vi "Fluke Calibrator.vi"(8 "error in (no error)":errorcluster, 11 "Fluke Calibrator in":refnum<class "Fluke Calibrator.lvclass">) -> (0 "error out":errorcluster, 3 "Fluke Calibrator out":refnum<class "Fluke Calibrator.lvclass">)   [LabVIEW 2012, in "Fluke Calibrator.lvclass"]
uses:
  Fluke Calibrator.lvclass
  Global/GPIB Numbers.vi
  Utility Classes/Readable/Readable.lvclass
panel:
  out "Status":string
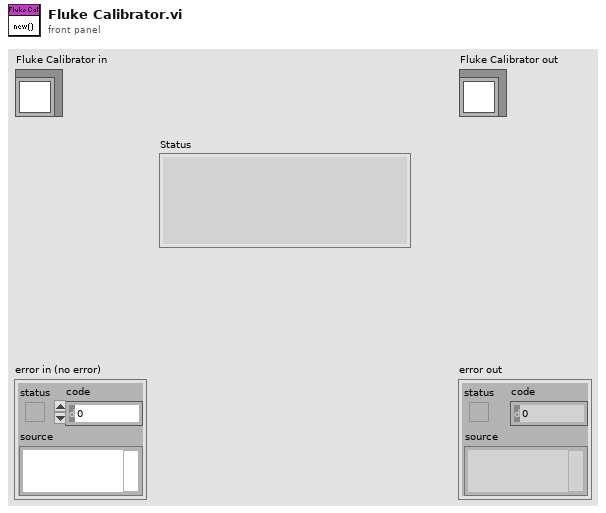
[diagram p1: front panel]
types:
  T1 = typedef "GPIB Type Def.ctl" = cluster{"Name":string, "bus":dbl, "GPIB":dbl, "GPIB as string":string, "byte":i32, "VISA Resource Name":refnum<visa-resource-name>}
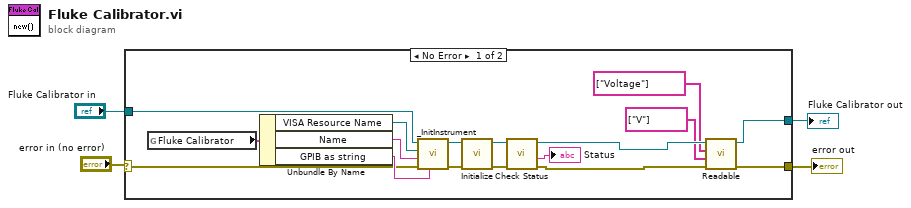
[diagram p0: block diagram]
diagram:
  n1 = case shown="No Error" "error in (no error)" {
    selector: "error in (no error)" -> [w16 w23]
    tunnel: [w14 w23] -> w2
    tunnel: [w11 w22] -> w1
    tunnel: "Fluke Calibrator in" -> [w20 w22]
    frame No Error {
      n2 = global read "GPIB Numbers.vi" "Fluke Calibrator"() -> (w21:T1)
      n3 = Unbundle By Name(w21) -> ("VISA Resource Name"=w19:refnum<visa-resource-name>, "Name"=w18:string, "GPIB as string"=w17:string)
      n4 = call-dynamic "_InitInstrument.vi"("GPIB as string"=w17, "error in (no error)"=w16, "Name"=w18, "VISA Resource Name"=w19, "Instrument in"=w20) -> ("error out"=w8:errorcluster, "Instrument out"=w7:refnum<class "Fluke Calibrator.lvclass">)  [unwired: 1 in, 4 out]
      n5 = call "Initialize.vi"("error in (no error)"=w8, "Fluke Calibrator in"=w7) -> ("error out"=w5:errorcluster, "Fluke Calibrator out"=w6:refnum<class "Fluke Calibrator.lvclass">)  [unwired: 8 in]
      n6 = call-dynamic "Check Status.vi"("error in (no error)"=w5, "Fluke Calibrator in"=w6) -> ("error out"=w13:errorcluster, "Status"=→"Status":string, "Fluke Calibrator out"=w12:refnum<class "Fluke Calibrator.lvclass">)  [unwired: 7 out]
      n7 = call "Readable.vi"("error in (no error)"=w13, "Channel Units"=string[] ["V"], "Channel Names"=string[] ["Voltage"], "Readable in"=w12) -> ("error out"=w14:errorcluster, "Readable out"=w11:refnum<class "Fluke Calibrator.lvclass">)  [unwired: 6 in]
    }
    frame Error {
    }
  }
  "error out" <- w2
  "Fluke Calibrator out" <- w1
